vi "eCapture.vi"() -> ()   [LabVIEW 2019]
uses:
  EmergentCameraC/EmergentCameraC.lvlib
panel:
  out "Height":u32
  out "Width":u32
  in  "FrameRate":u32(slide) min=1 max=35 step=1 scale=1.0..35.0
  in  "Exposure":u32(slide) min=1 max=28116 step=1 scale=1.0..28116.0
  out "Image":T1(plugin-control)
  in  "OnOff":bool
  out "PixelFormat":string
  out "Vendor":string
  out "ip":string
  out "Version":string
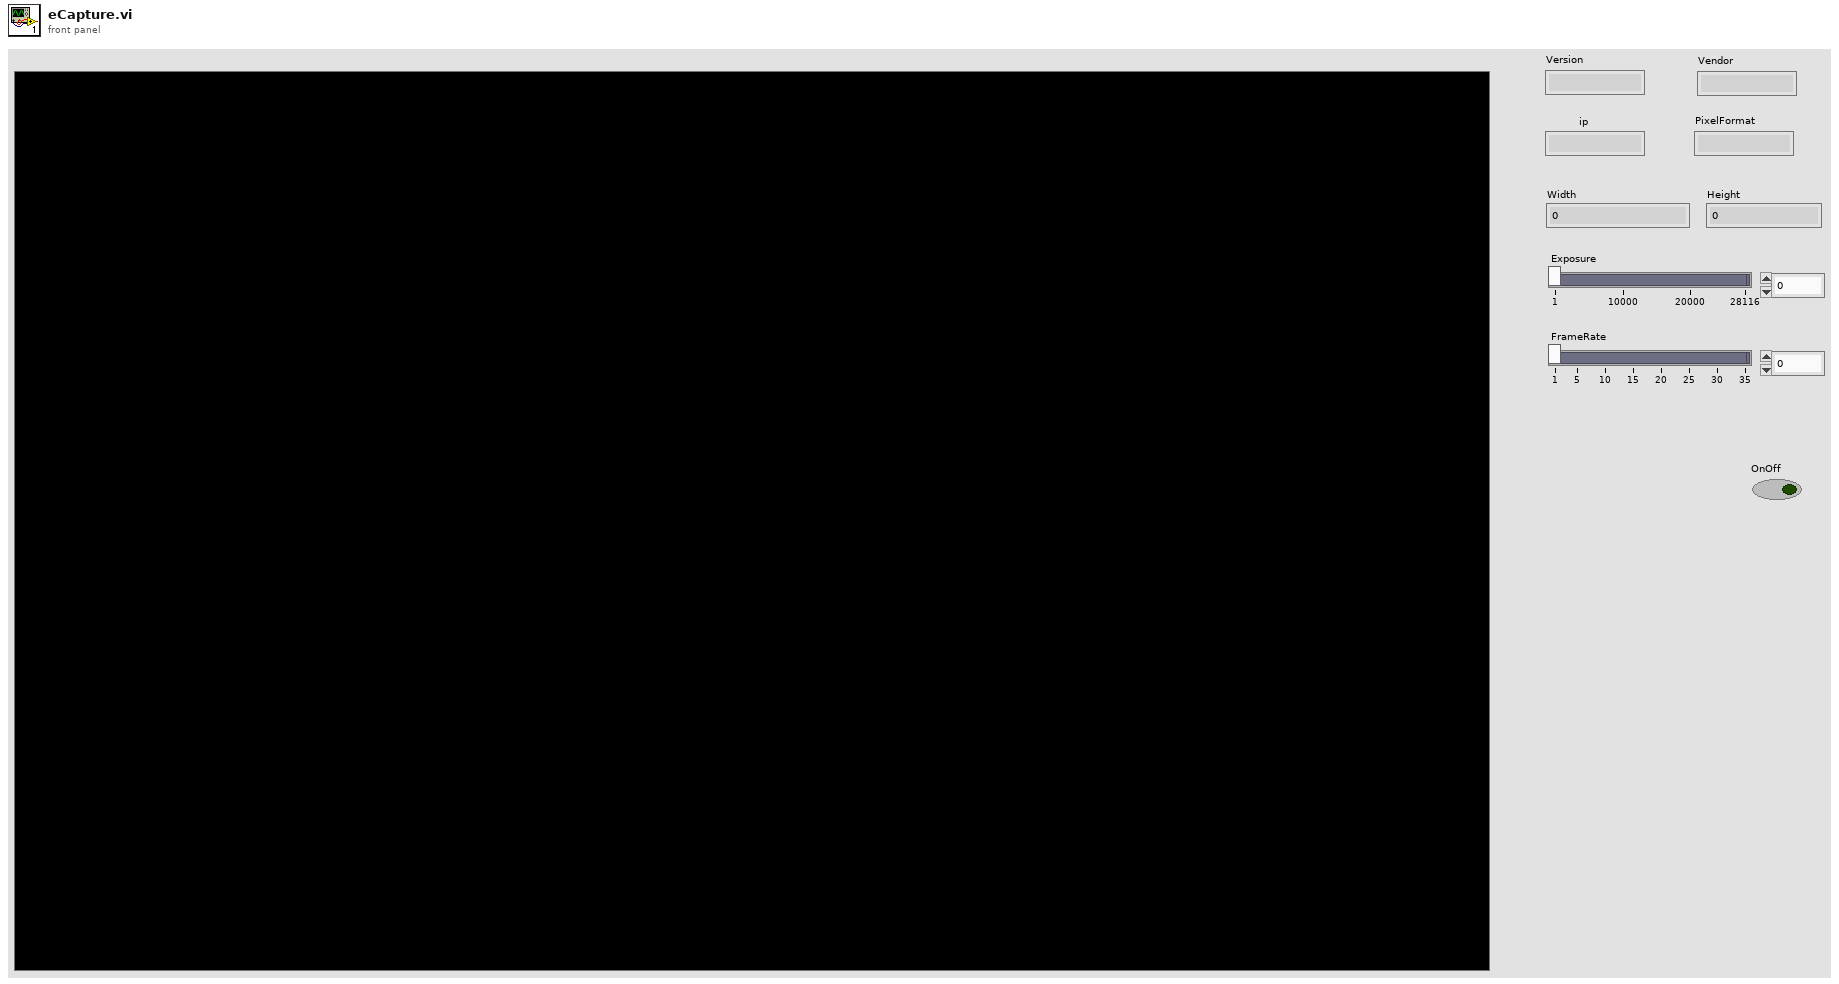
[diagram p1: front panel]
types:
  T1 = typedef "IMAQ Image.ctl" = refnum<image>
  T2 = enum8{"Enabled", "Disabled", "Disabled and Grayed Out"}
  T3 = cluster{"specVersionMajor":u16, "specVersionMinor":u16, "deviceMode":u32, "macAddress[0]":i8, "macAddress[1]":i8, "macAddress[2]":i8, "macAddress[3]":i8, "macAddress[4]":i8, "macAddress[5]":i8, "macAddress[6]":i8, "macAddress[7]":i8, "macAddress[8]":i8, "macAddress[9]":i8, "macAddress[10]":i8, "macAddress[11]":i8, "macAddress[12]":i8, "macAddress[13]":i8, "macAddress[14]":i8, "macAddress[15]":i8, "macAddress[16]":i8, "macAddress[17]":i8, "@dummy control@":i8, "@dummy control@":i8, "ipConfigOptions":u32, "ipConfigCurrent":u32, "currentIp[0]":i8, "currentIp[1]":i8, "currentIp[2]":i8, "currentIp[3]":i8, "currentIp[4]":i8, "currentIp[5]":i8, "currentIp[6]":i8, "currentIp[7]":i8, "currentIp[8]":i8, "currentIp[9]":i8, "currentIp[10]":i8, "currentIp[11]":i8, "currentIp[12]":i8, "currentIp[13]":i8, "currentIp[14]":i8, "currentIp[15]":i8, "currentSubnetMask[0]":i8, "currentSubnetMask[1]":i8, "currentSubnetMask[2]":i8, "currentSubnetMask[3]":i8, "currentSubnetMask[4]":i8, "currentSubnetMask[5]":i8, "currentSubnetMask[6]":i8, "currentSubnetMask[7]":i8, "currentSubnetMask[8]":i8, "currentSubnetMask[9]":i8, "currentSubnetMask[10]":i8, "currentSubnetMask[11]":i8, "currentSubnetMask[12]":i8, "currentSubnetMask[13]":i8, "currentSubnetMask[14]":i8, "currentSubnetMask[15]":i8, "defaultGateway[0]":i8, "defaultGateway[1]":i8, "defaultGateway[2]":i8, "defaultGateway[3]":i8, "defaultGateway[4]":i8, "defaultGateway[5]":i8, "defaultGateway[6]":i8, "defaultGateway[7]":i8, "defaultGateway[8]":i8, "defaultGateway[9]":i8, "defaultGateway[10]":i8, "defaultGateway[11]":i8, "defaultGateway[12]":i8, "defaultGateway[13]":i8, "defaultGateway[14]":i8, "defaultGateway[15]":i8, "manufacturerName[0]":i8, "manufacturerName[1]":i8, "manufacturerName[2]":i8, "manufacturerName[3]":i8, "manufacturerName[4]":i8, "manufacturerName[5]":i8, "manufacturerName[6]":i8, "manufacturerName[7]":i8, "manufacturerName[8]":i8, "manufacturerName[9]":i8, "manufacturerName[10]":i8, "manufacturerName[11]":i8, "manufacturerName[12]":i8, "manufacturerName[13]":i8, "manufacturerName[14]":i8, "manufacturerName[15]":i8, "manufacturerName[16]":i8, "manufacturerName[17]":i8, "manufacturerName[18]":i8, "manufacturerName[19]":i8, "manufacturerName[20]":i8, "manufacturerName[21]":i8, "manufacturerName[22]":i8, "manufacturerName[23]":i8, "manufacturerName[24]":i8, "manufacturerName[25]":i8, "manufacturerName[26]":i8, "manufacturerName[27]":i8, "manufacturerName[28]":i8, "manufacturerName[29]":i8, "manufacturerName[30]":i8, "manufacturerName[31]":i8, "modelName[0]":i8, "modelName[1]":i8, "modelName[2]":i8, "modelName[3]":i8, "modelName[4]":i8, "modelName[5]":i8, "modelName[6]":i8, "modelName[7]":i8, "modelName[8]":i8, "modelName[9]":i8, "modelName[10]":i8, "modelName[11]":i8, "modelName[12]":i8, "modelName[13]":i8, "modelName[14]":i8, "modelName[15]":i8, "modelName[16]":i8, "modelName[17]":i8, "modelName[18]":i8, "modelName[19]":i8, "modelName[20]":i8, "modelName[21]":i8, "modelName[22]":i8, "modelName[23]":i8, "modelName[24]":i8, "modelName[25]":i8, "modelName[26]":i8, "modelName[27]":i8, "modelName[28]":i8, "modelName[29]":i8, "modelName[30]":i8, "modelName[31]":i8, "deviceVersion[0]":i8, "deviceVersion[1]":i8, "deviceVersion[2]":i8, "deviceVersion[3]":i8, "deviceVersion[4]":i8, "deviceVersion[5]":i8, "deviceVersion[6]":i8, "deviceVersion[7]":i8, "deviceVersion[8]":i8, "deviceVersion[9]":i8, "deviceVersion[10]":i8, "deviceVersion[11]":i8, "deviceVersion[12]":i8, "deviceVersion[13]":i8, "deviceVersion[14]":i8, "deviceVersion[15]":i8, "deviceVersion[16]":i8, "deviceVersion[17]":i8, "deviceVersion[18]":i8, "deviceVersion[19]":i8, "deviceVersion[20]":i8, "deviceVersion[21]":i8, "deviceVersion[22]":i8, "deviceVersion[23]":i8, "deviceVersion[24]":i8, "deviceVersion[25]":i8, "deviceVersion[26]":i8, "deviceVersion[27]":i8, "deviceVersion[28]":i8, "deviceVersion[29]":i8, "deviceVersion[30]":i8, "deviceVersion[31]":i8, "manufacturerSpecifiedInfo[0]":i8, "manufacturerSpecifiedInfo[1]":i8, "manufacturerSpecifiedInfo[2]":i8, "manufacturerSpecifiedInfo[3]":i8, "manufacturerSpecifiedInfo[4]":i8, "manufacturerSpecifiedInfo[5]":i8, "manufacturerSpecifiedInfo[6]":i8, "manufacturerSpecifiedInfo[7]":i8, "manufacturerSpecifiedInfo[8]":i8, "manufacturerSpecifiedInfo[9]":i8, "manufacturerSpecifiedInfo[10]":i8, "manufacturerSpecifiedInfo[11]":i8, "manufacturerSpecifiedInfo[12]":i8, "manufacturerSpecifiedInfo[13]":i8, "manufacturerSpecifiedInfo[14]":i8, "manufacturerSpecifiedInfo[15]":i8, "manufacturerSpecifiedInfo[16]":i8, "manufacturerSpecifiedInfo[17]":i8, "manufacturerSpecifiedInfo[18]":i8, "manufacturerSpecifiedInfo[19]":i8, "manufacturerSpecifiedInfo[20]":i8, "manufacturerSpecifiedInfo[21]":i8, "manufacturerSpecifiedInfo[22]":i8, "manufacturerSpecifiedInfo[23]":i8, "manufacturerSpecifiedInfo[24]":i8, "manufacturerSpecifiedInfo[25]":i8, "manufacturerSpecifiedInfo[26]":i8, "manufacturerSpecifiedInfo[27]":i8, "manufacturerSpecifiedInfo[28]":i8, "manufacturerSpecifiedInfo[29]":i8, "manufacturerSpecifiedInfo[30]":i8, "manufacturerSpecifiedInfo[31]":i8, "manufacturerSpecifiedInfo[32]":i8, "manufacturerSpecifiedInfo[33]":i8, "manufacturerSpecifiedInfo[34]":i8, "manufacturerSpecifiedInfo[35]":i8, "manufacturerSpecifiedInfo[36]":i8, "manufacturerSpecifiedInfo[37]":i8, "manufacturerSpecifiedInfo[38]":i8, "manufacturerSpecifiedInfo[39]":i8, "manufacturerSpecifiedInfo[40]":i8, "manufacturerSpecifiedInfo[41]":i8, "manufacturerSpecifiedInfo[42]":i8, "manufacturerSpecifiedInfo[43]":i8, "manufacturerSpecifiedInfo[44]":i8, "manufacturerSpecifiedInfo[45]":i8, "manufacturerSpecifiedInfo[46]":i8, "manufacturerSpecifiedInfo[47]":i8, "serialNumber[0]":i8, "serialNumber[1]":i8, "serialNumber[2]":i8, "serialNumber[3]":i8, "serialNumber[4]":i8, "serialNumber[5]":i8, "serialNumber[6]":i8, "serialNumber[7]":i8, "serialNumber[8]":i8, "serialNumber[9]":i8, "serialNumber[10]":i8, "serialNumber[11]":i8, "serialNumber[12]":i8, "serialNumber[13]":i8, "serialNumber[14]":i8, "serialNumber[15]":i8, "userDefinedName[0]":i8, "userDefinedName[1]":i8, "userDefinedName[2]":i8, "userDefinedName[3]":i8, "userDefinedName[4]":i8, "userDefinedName[5]":i8, "userDefinedName[6]":i8, "userDefinedName[7]":i8, "userDefinedName[8]":i8, "userDefinedName[9]":i8, "userDefinedName[10]":i8, "userDefinedName[11]":i8, "userDefinedName[12]":i8, "userDefinedName[13]":i8, "userDefinedName[14]":i8, "userDefinedName[15]":i8, "ip4Address[0]":i8, "ip4Address[1]":i8, "ip4Address[2]":i8, "ip4Address[3]":i8, "ip4Address[4]":i8, "ip4Address[5]":i8, "ip4Address[6]":i8, "ip4Address[7]":i8, "ip4Address[8]":i8, "ip4Address[9]":i8, "ip4Address[10]":i8, "ip4Address[11]":i8, "ip4Address[12]":i8, "ip4Address[13]":i8, "ip4Address[14]":i8, "ip4Address[15]":i8, "ip4AddressBroadcast[0]":i8, "ip4AddressBroadcast[1]":i8, "ip4AddressBroadcast[2]":i8, "ip4AddressBroadcast[3]":i8, "ip4AddressBroadcast[4]":i8, "ip4AddressBroadcast[5]":i8, "ip4AddressBroadcast[6]":i8, "ip4AddressBroadcast[7]":i8, "ip4AddressBroadcast[8]":i8, "ip4AddressBroadcast[9]":i8, "ip4AddressBroadcast[10]":i8, "ip4AddressBroadcast[11]":i8, "ip4AddressBroadcast[12]":i8, "ip4AddressBroadcast[13]":i8, "ip4AddressBroadcast[14]":i8, "ip4AddressBroadcast[15]":i8, "friendlyName[0]":i8, "friendlyName[1]":i8, "friendlyName[2]":i8, "friendlyName[3]":i8, "friendlyName[4]":i8, "friendlyName[5]":i8, "friendlyName[6]":i8, "friendlyName[7]":i8, "friendlyName[8]":i8, "friendlyName[9]":i8, "friendlyName[10]":i8, "friendlyName[11]":i8, "friendlyName[12]":i8, "friendlyName[13]":i8, "friendlyName[14]":i8, "friendlyName[15]":i8, "friendlyName[16]":i8, "friendlyName[17]":i8, "friendlyName[18]":i8, "friendlyName[19]":i8, "friendlyName[20]":i8, "friendlyName[21]":i8, "friendlyName[22]":i8, "friendlyName[23]":i8, "friendlyName[24]":i8, "friendlyName[25]":i8, "friendlyName[26]":i8, "friendlyName[27]":i8, "friendlyName[28]":i8, "friendlyName[29]":i8, "friendlyName[30]":i8, "friendlyName[31]":i8, "friendlyName[32]":i8, "friendlyName[33]":i8, "friendlyName[34]":i8, "friendlyName[35]":i8, "friendlyName[36]":i8, "friendlyName[37]":i8, "friendlyName[38]":i8, "friendlyName[39]":i8, "friendlyName[40]":i8, "friendlyName[41]":i8, "friendlyName[42]":i8, "friendlyName[43]":i8, "friendlyName[44]":i8, "friendlyName[45]":i8, "friendlyName[46]":i8, "friendlyName[47]":i8, "friendlyName[48]":i8, "friendlyName[49]":i8, "friendlyName[50]":i8, "friendlyName[51]":i8, "friendlyName[52]":i8, "friendlyName[53]":i8, "friendlyName[54]":i8, "friendlyName[55]":i8, "friendlyName[56]":i8, "friendlyName[57]":i8, "friendlyName[58]":i8, "friendlyName[59]":i8, "friendlyName[60]":i8, "friendlyName[61]":i8, "friendlyName[62]":i8, "friendlyName[63]":i8, "friendlyName[64]":i8, "friendlyName[65]":i8, "friendlyName[66]":i8, "friendlyName[67]":i8, "friendlyName[68]":i8, "friendlyName[69]":i8, "friendlyName[70]":i8, "friendlyName[71]":i8, "friendlyName[72]":i8, "friendlyName[73]":i8, "friendlyName[74]":i8, "friendlyName[75]":i8, "friendlyName[76]":i8, "friendlyName[77]":i8, "friendlyName[78]":i8, "friendlyName[79]":i8, "friendlyName[80]":i8, "friendlyName[81]":i8, "friendlyName[82]":i8, "friendlyName[83]":i8, "friendlyName[84]":i8, "friendlyName[85]":i8, "friendlyName[86]":i8, "friendlyName[87]":i8, "friendlyName[88]":i8, "friendlyName[89]":i8, "friendlyName[90]":i8, "friendlyName[91]":i8, "friendlyName[92]":i8, "friendlyName[93]":i8, "friendlyName[94]":i8, "friendlyName[95]":i8, "friendlyName[96]":i8, "friendlyName[97]":i8, "friendlyName[98]":i8, "friendlyName[99]":i8, "friendlyName[100]":i8, "friendlyName[101]":i8, "friendlyName[102]":i8, "friendlyName[103]":i8, "friendlyName[104]":i8, "friendlyName[105]":i8, "friendlyName[106]":i8, "friendlyName[107]":i8, "friendlyName[108]":i8, "friendlyName[109]":i8, "friendlyName[110]":i8, "friendlyName[111]":i8, "friendlyName[112]":i8, "friendlyName[113]":i8, "friendlyName[114]":i8, "friendlyName[115]":i8, "friendlyName[116]":i8, "friendlyName[117]":i8, "friendlyName[118]":i8, "friendlyName[119]":i8, "friendlyName[120]":i8, "friendlyName[121]":i8, "friendlyName[122]":i8, "friendlyName[123]":i8, "friendlyName[124]":i8, "friendlyName[125]":i8, "friendlyName[126]":i8, "friendlyName[127]":i8, "description[0]":i8, "description[1]":i8, "description[2]":i8, "description[3]":i8, "description[4]":i8, "description[5]":i8, "description[6]":i8, "description[7]":i8, "description[8]":i8, "description[9]":i8, "description[10]":i8, "description[11]":i8, "description[12]":i8, "description[13]":i8, "description[14]":i8, "description[15]":i8, "description[16]":i8, "description[17]":i8, "description[18]":i8, "description[19]":i8, "description[20]":i8, "description[21]":i8, "description[22]":i8, "description[23]":i8, "description[24]":i8, "description[25]":i8, "description[26]":i8, "description[27]":i8, "description[28]":i8, "description[29]":i8, "description[30]":i8, "description[31]":i8, "description[32]":i8, "description[33]":i8, "description[34]":i8, "description[35]":i8, "description[36]":i8, "description[37]":i8, "description[38]":i8, "description[39]":i8, "description[40]":i8, "description[41]":i8, "description[42]":i8, "description[43]":i8, "description[44]":i8, "description[45]":i8, "description[46]":i8, "description[47]":i8, "description[48]":i8, "description[49]":i8, "description[50]":i8, "description[51]":i8, "description[52]":i8, "description[53]":i8, "description[54]":i8, "description[55]":i8, "description[56]":i8, "description[57]":i8, "description[58]":i8, "description[59]":i8, "description[60]":i8, "description[61]":i8, "description[62]":i8, "description[63]":i8, "description[64]":i8, "description[65]":i8, "description[66]":i8, "description[67]":i8, "description[68]":i8, "description[69]":i8, "description[70]":i8, "description[71]":i8, "description[72]":i8, "description[73]":i8, "description[74]":i8, "description[75]":i8, "description[76]":i8, "description[77]":i8, "description[78]":i8, "description[79]":i8, "description[80]":i8, "description[81]":i8, "description[82]":i8, "description[83]":i8, "description[84]":i8, "description[85]":i8, "description[86]":i8, "description[87]":i8, "description[88]":i8, "description[89]":i8, "description[90]":i8, "description[91]":i8, "description[92]":i8, "description[93]":i8, "description[94]":i8, "description[95]":i8, "description[96]":i8, "description[97]":i8, "description[98]":i8, "description[99]":i8, "description[100]":i8, "description[101]":i8, "description[102]":i8, "description[103]":i8, "description[104]":i8, "description[105]":i8, "description[106]":i8, "description[107]":i8, "description[108]":i8, "description[109]":i8, "description[110]":i8, "description[111]":i8, "description[112]":i8, "description[113]":i8, "description[114]":i8, "description[115]":i8, "description[116]":i8, "description[117]":i8, "description[118]":i8, "description[119]":i8, "description[120]":i8, "description[121]":i8, "description[122]":i8, "description[123]":i8, "description[124]":i8, "description[125]":i8, "description[126]":i8, "description[127]":i8, "adapterName[0]":i8, "adapterName[1]":i8, "adapterName[2]":i8, "adapterName[3]":i8, "adapterName[4]":i8, "adapterName[5]":i8, "adapterName[6]":i8, "adapterName[7]":i8, "adapterName[8]":i8, "adapterName[9]":i8, "adapterName[10]":i8, "adapterName[11]":i8, "adapterName[12]":i8, "adapterName[13]":i8, "adapterName[14]":i8, "adapterName[15]":i8, "adapterName[16]":i8, "adapterName[17]":i8, "adapterName[18]":i8, "adapterName[19]":i8, "adapterName[20]":i8, "adapterName[21]":i8, "adapterName[22]":i8, "adapterName[23]":i8, "adapterName[24]":i8, "adapterName[25]":i8, "adapterName[26]":i8, "adapterName[27]":i8, "adapterName[28]":i8, "adapterName[29]":i8, "adapterName[30]":i8, "adapterName[31]":i8, "adapterName[32]":i8, "adapterName[33]":i8, "adapterName[34]":i8, "adapterName[35]":i8, "adapterName[36]":i8, "adapterName[37]":i8, "adapterName[38]":i8, "adapterName[39]":i8, "adapterName[40]":i8, "adapterName[41]":i8, "adapterName[42]":i8, "adapterName[43]":i8, "adapterName[44]":i8, "adapterName[45]":i8, "adapterName[46]":i8, "adapterName[47]":i8, "adapterName[48]":i8, "adapterName[49]":i8, "adapterName[50]":i8, "adapterName[51]":i8, "adapterName[52]":i8, "adapterName[53]":i8, "adapterName[54]":i8, "adapterName[55]":i8, "adapterName[56]":i8, "adapterName[57]":i8, "adapterName[58]":i8, "adapterName[59]":i8, "adapterName[60]":i8, "adapterName[61]":i8, "adapterName[62]":i8, "adapterName[63]":i8, "adapterName[64]":i8, "adapterName[65]":i8, "adapterName[66]":i8, "adapterName[67]":i8, "adapterName[68]":i8, "adapterName[69]":i8, "adapterName[70]":i8, "adapterName[71]":i8, "adapterName[72]":i8, "adapterName[73]":i8, "adapterName[74]":i8, "adapterName[75]":i8, "adapterName[76]":i8, "adapterName[77]":i8, "adapterName[78]":i8, "adapterName[79]":i8, "adapterName[80]":i8, "adapterName[81]":i8, "adapterName[82]":i8, "adapterName[83]":i8, "adapterName[84]":i8, "adapterName[85]":i8, "adapterName[86]":i8, "adapterName[87]":i8, "adapterName[88]":i8, "adapterName[89]":i8, "adapterName[90]":i8, "adapterName[91]":i8, "adapterName[92]":i8, "adapterName[93]":i8, "adapterName[94]":i8, "adapterName[95]":i8, "adapterName[96]":i8, "adapterName[97]":i8, "adapterName[98]":i8, "adapterName[99]":i8, "adapterName[100]":i8, "adapterName[101]":i8, "adapterName[102]":i8, "adapterName[103]":i8, "adapterName[104]":i8, "adapterName[105]":i8, "adapterName[106]":i8, "adapterName[107]":i8, "adapterName[108]":i8, "adapterName[109]":i8, "adapterName[110]":i8, "adapterName[111]":i8, "adapterName[112]":i8, "adapterName[113]":i8, "adapterName[114]":i8, "adapterName[115]":i8, "adapterName[116]":i8, "adapterName[117]":i8, "adapterName[118]":i8, "adapterName[119]":i8, "adapterName[120]":i8, "adapterName[121]":i8, "adapterName[122]":i8, "adapterName[123]":i8, "adapterName[124]":i8, "adapterName[125]":i8, "adapterName[126]":i8, "adapterName[127]":i8, "vendorID":u32, "@dummy control@":i8, "@dummy control@":i8, "@dummy control@":i8, "@dummy control@":i8, "@dummy control@":i8, "@dummy control@":i8, "@dummy control@":i8, "@dummy control@":i8, "name":u64, "fullName":u64, "mtu":u32}
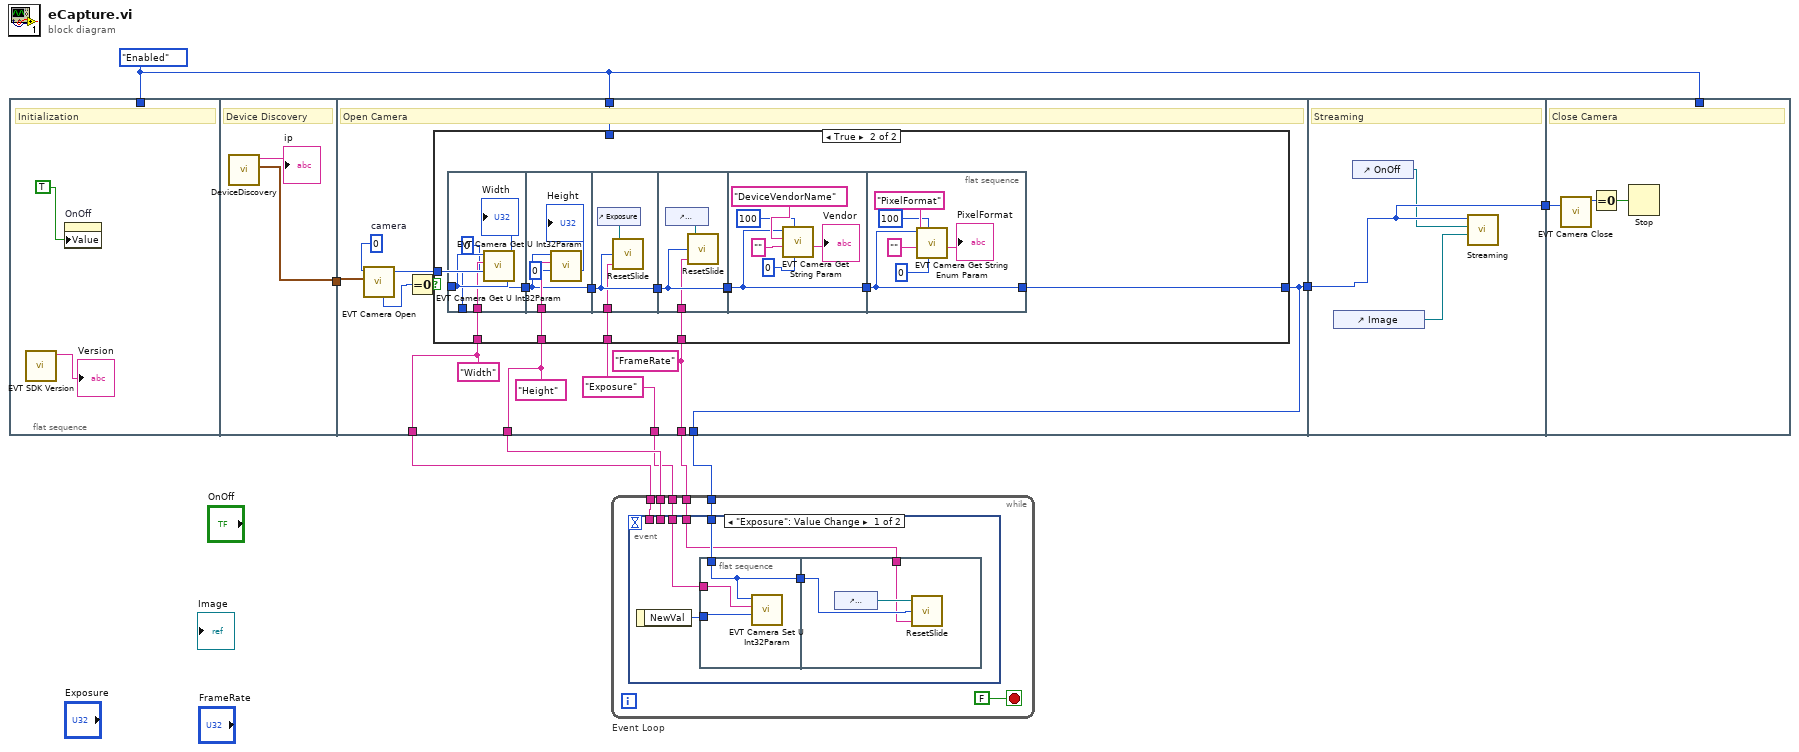
[diagram p0: block diagram]
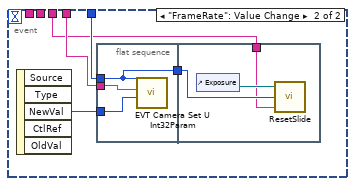
[diagram p2: hidden frame]
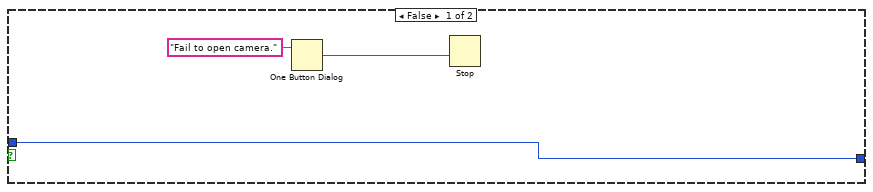
[diagram p3: hidden frame]
diagram:
  w2 = T2."Enabled" ("Disabled")
  n1 = flat-sequence {
    tunnel: w2 -> [_]
    tunnel: [w12] -> w1
    tunnel: [w19] -> w9
    tunnel: [w21] -> w7
    tunnel: [w19] -> w8
    tunnel: [w20] -> w6
    tunnel: [w18] -> w4
    tunnel: [w17] -> w3
    tunnel: w2 -> [w16]
    tunnel: w1 -> [w14]
    tunnel: w9 -> [w67]
    tunnel: [w67] -> w5
    tunnel: w5 -> [w69]
    tunnel: w2 -> [_]
    frame #0 {
      # "Initialization"
      n2 = call "EVT SDK Version.vi"() -> ("function return"=→"Version":string)  [unwired: 11 in]
      n3 = property on="OnOff" class="Bool (strict)"("Value"=TRUE ("Display Image")) -> ()  [unwired: 2 in, 2 out]
    }
    frame #1 {
      # "Device Discovery"
      n4 = call "DeviceDiscovery.vi"() -> ("deviceInfo out"=w12:T3, "Ip"=→"ip":string)  [unwired: 10 in]
    }
    frame #2 {
      w17 = "FrameRate"
      w18 = "Exposure"
      w20 = "Height"
      w21 = "Width"
      w23 = u64 0  # camera
      # "Open Camera"
      n5 = call "EVT Camera Open.vi"("deviceInfo"=w14, "cameraHandle"=w23) -> ("cameraHandle out"=w24:u64, "function return"=w15:u32)  [unwired: 5 in, 3 out]
      n6 = Equal To 0?(x=w15) -> (x = 0?=w22:bool)
      n7 = case shown="True" w22 {
        tunnel: w24 -> [w25 w38]
        tunnel: w21 -> [_ w36]
        tunnel: w20 -> [_ w35]
        tunnel: [w25 w34] -> w19
        tunnel: w18 -> [_ w32]
        tunnel: w17 -> [_ w30]
        tunnel: w16 -> [_ _]
        frame False {
          n8 = One Button Dialog(message="Fail to open camera.") -> (true=w26:bool)  [unwired: 1 in]
          n9 = Stop(stop? (T)=w26) -> ()
        }
        frame True {
          n10 = flat-sequence {
            tunnel: w38 -> [w42]
            tunnel: w36 -> [w41]
            tunnel: [w42] -> w37
            tunnel: [w39] -> _
            tunnel: w37 -> [w45]
            tunnel: w35 -> [w46]
            tunnel: [w45] -> w28
            tunnel: w28 -> [w48]
            tunnel: [w48] -> w31
            tunnel: w32 -> [w47]
            tunnel: w31 -> [w51]
            tunnel: [w51] -> w29
            tunnel: w30 -> [w50]
            tunnel: w29 -> [w54]
            tunnel: [w54] -> w33
            tunnel: [w61] -> w34
            tunnel: w33 -> [w61]
            frame #0 {
              n11 = call "EVT Camera Get U Int32Param.vi"("val"=u32 0, "name"=w41, "camera"=w42) -> ("val out"=w39:u32)  [unwired: 7 in, 1 out]
              "Width" <- w39
            }
            frame #1 {
              n12 = call "EVT Camera Get U Int32Param.vi"("val"=u32 0, "name"=w46, "camera"=w45) -> ("val out"=→"Height":u32)  [unwired: 7 in, 1 out]
            }
            frame #2 {
              n13 = control-ref of="Exposure"() -> (w49:refnum<vi>)
              n14 = call "ResetSlide.vi"("name"=w47, "camera"=w48, "SlideRef"=w49) -> ()  [unwired: 1 in]
            }
            frame #3 {
              n15 = control-ref of="FrameRate"() -> (w52:refnum<vi>)
              n16 = call "ResetSlide.vi"("name"=w50, "camera"=w51, "SlideRef"=w52) -> ()  [unwired: 1 in]
            }
            frame #4 {
              n17 = call "EVT Camera Get String Param.vi"("valueSize"=u32 0 ("bufferSize"), "bufferSize"=u32 100, "buffer"="", "name"="DeviceVendorName", "camera"=w54) -> ("buffer out"=→"Vendor":string)  [unwired: 4 in, 2 out]
            }
            frame #5 {
              n18 = call "EVT Camera Get String Enum Param.vi"("valueSize"=u32 0, "bufferSize"=u32 100, "buffer"="", "name"="PixelFormat", "camera"=w61) -> ("buffer out"=→"PixelFormat":string)  [unwired: 4 in, 2 out]
            }
          }
        }
      }
    }
    frame #3 {
      # "Streaming"
      n19 = control-ref of="Image"() -> (w65:refnum<vi>)
      n20 = control-ref of="OnOff"() -> (w66:refnum<vi>)
      n21 = call "Streaming.vi"("Image Display Refnum"=w65, "OnOff Refnum"=w66, "camera"=w67) -> ()  [unwired: 9 in]
    }
    frame #4 {
      # "Close Camera"
      n22 = call "EVT Camera Close.vi"("cameraHandle"=w69) -> ("function return"=w68:u32)  [unwired: 10 in]
      n23 = Equal To 0?(x=w68) -> (x = 0?=w70:bool)
      n24 = Stop(stop? (T)=w70) -> ()
    }
  }
  n25 = while "Event Loop" {
    tunnel: w8 -> [w76]
    tunnel: w7 -> [w75]
    tunnel: w6 -> [w73]
    tunnel: w4 -> [w72]
    tunnel: w3 -> [w71]
    stop <- FALSE stop-if-true
    n26 = event shown="[0] \"Exposure\": Value Change" {
      selector: _ -> [_ _]
      dyn-events: _ -> [_ _]
      timeout: _ -> [_ _]
      tunnel: w76 -> [w79 w90]
      tunnel: w75 -> [_ _]
      tunnel: w73 -> [_ _]
      tunnel: w72 -> [w81 w88]
      tunnel: w71 -> [w77 w91]
      event "Exposure": Value Change {
        n27 = event-data() -> ("NewVal"=w80:u32)  [unwired: 1 in]
        n28 = flat-sequence {
          tunnel: w81 -> [w84]
          tunnel: w80 -> [w83]
          tunnel: w79 -> [w82]
          tunnel: [w82] -> w78
          tunnel: w78 -> [w86]
          tunnel: w77 -> [w85]
          frame #0 {
            n29 = call "EVT Camera Set U Int32Param.vi"("val"=w83, "name"=w84, "camera"=w82) -> ()  [unwired: 8 in, 1 out]
          }
          frame #1 {
            n30 = control-ref of="FrameRate"() -> (w87:refnum<vi>)
            n31 = call "ResetSlide.vi"("name"=w85, "camera"=w86, "SlideRef"=w87) -> ()  [unwired: 1 in]
          }
        }
      }
      event "FrameRate": Value Change {
        n32 = event-data() -> ("NewVal"=w92:u32)  [unwired: 1 in, 4 out]
        n33 = flat-sequence {
          tunnel: w92 -> [w94]
          tunnel: w91 -> [w95]
          tunnel: w90 -> [w93]
          tunnel: [w93] -> w89
          tunnel: w89 -> [w97]
          tunnel: w88 -> [w96]
          frame #0 {
            n34 = call "EVT Camera Set U Int32Param.vi"("val"=w94, "name"=w95, "camera"=w93) -> ()  [unwired: 8 in, 1 out]
          }
          frame #1 {
            n35 = control-ref of="Exposure"() -> (w98:refnum<vi>)
            n36 = call "ResetSlide.vi"("name"=w96, "camera"=w97, "SlideRef"=w98) -> ()  [unwired: 1 in]
          }
        }
      }
    }
  }
